vi "Read Measurement name.vi"(8 "error in (no error)":errorcluster, 11 "Mag Lab Measurement in":refnum<class "Mag Lab Measurement.lvclass">) -> (0 "error out":errorcluster, 2 "Measurement name":string, 3 "Mag Lab Measurement out":refnum<class "Mag Lab Measurement.lvclass">)   [LabVIEW 2015, in "Mag Lab Measurement.lvclass"]
uses:
  Mag Lab Measurement.lvclass
  Mag Lab Measurement.lvclass/Mag Lab Measurement.ctl
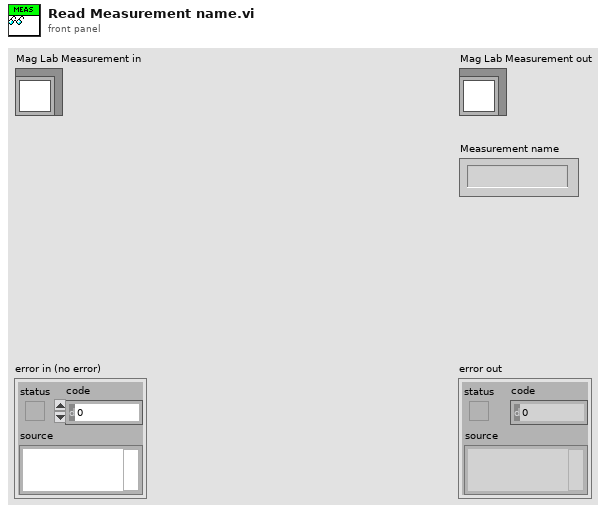
[diagram p1: front panel]
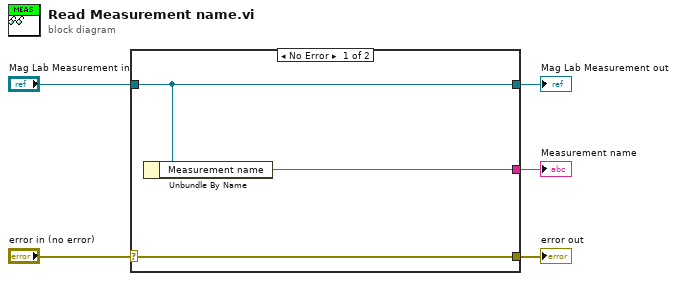
[diagram p0: block diagram]
diagram:
  n1 = case shown="No Error" "error in (no error)" {
    selector: "error in (no error)" -> [w8 w9]
    tunnel: [w8 w9] -> w4
    tunnel: [w7 w10] -> w2
    tunnel: "Mag Lab Measurement in" -> [w7 w10]
    tunnel: [w6 _] -> w1
    frame No Error {
      n2 = Unbundle By Name(w7) -> ("Measurement name"=w6:string)
    }
    frame Error {
    }
  }
  "error out" <- w4
  "Mag Lab Measurement out" <- w2
  "Measurement name" <- w1
